vi "solar_qtimer Set (EnQType).vi"(8 "error in (no error)":errorcluster, 10 "EnQ_Type (IgnoreIfExists)":enum8{"Normal", "Priority", "IgnoreIfExists"}(ring)=enum."IgnoreIfExists", 11 "QTimer Name":string) -> (0 "error out":errorcluster)   [LabVIEW 2018]
doc: "[DEPRECIATED] This sets the enqueue type of the QTimer by name.\nIgnore If Exists: Does not enqueue the command if it already exists in the queue\nNormal: Always enqueues a new message\nPriority: Enqueues the message on the front of the queue."
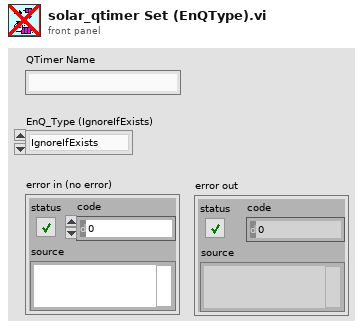
[diagram p1: front panel]
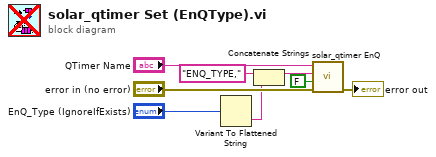
[diagram p0: block diagram]
diagram:
  n1 = Variant To Flattened String(Variant="EnQ_Type (IgnoreIfExists)") -> (data string=w3:string)  [unwired: 1 out]
  n2 = Concatenate Strings("ENQ_TYPE," ("CMD (\"\")"), w3) -> (w4:string)
  n3 = call "solar_qtimer EnQ.vi"("error in (no error)"="error in (no error)", "Create if not found? (F)"=FALSE, "CMD (\"\")"=w4, "QTimer Name"="QTimer Name") -> ("error out"=→"error out":errorcluster)  [unwired: 5 in, 2 out]
